vi "TrendPlot.vi"(6 "Zen Analytics in":refnum<class "Zen Analytics.lvclass">, 8 "error in (no error)":errorcluster, 9 "Graph Refference's":T2, 10 "IndexOfMeasurement":i32, 11 "Plot Cluster":T1) -> (0 "error out":errorcluster)   [LabVIEW 2019, in "Zen Analytics.lvlib" / "Zen Analytics.lvclass"]
uses:
  Zen Analytics.lvclass
  Dependency/GraphReff.ctl
  Dependency/Plot Cluster.ctl
types:
  T1 = typedef "Zen Analytics.lvlib/Zen Analytics.lvclass/Plot Cluster.ctl" = cluster{"Reduced 2D":dbl[][], "Start Index":i32, "No Of New Termnals":i32, "Top/Bottom":bool, "Values Inserted":i32, "Re-Initialised":bool, "Statistical params":string[][], "MeasurementInitializationData":cluster{"Measurement-ID":i32[], "Measurement Names":string[], "NominalValues":dbl[], "LSL":dbl[], "USL":dbl[], "LCL":dbl[], "UCL":dbl[]}, "MeasurementData":cluster{"Measurement ID":i32, "Measurement Name":string, "Nominal Values":dbl, "LSL":dbl, "USL":dbl, "LCL":dbl, "UCL":dbl}[], "ResultData2D":dbl[][], "PlotParameters":cluster{"Trend":cluster{"TrendPlotID":dbl, "PlotProperties":cluster{"FontName":string, "FontSize":dbl, "FontColor":string, "IsBold":bool, "IsItalic":bool, "PlotColor":string}}[], "Histogram":cluster{"HistogramPlotID":dbl, "PlotProperties":cluster{"FontName":string, "FontSize":dbl, "FontColor":string, "IsBold":bool, "IsItalic":bool, "PlotColor":string}}[], "BarPlot":cluster{"BarPlotID":dbl, "BarValuesID":dbl, "PlotProperties":cluster{"FontName":string, "FontSize":dbl, "IsBold":bool, "IsItalic":bool, "FontColor":string}, "Sectors":string[]}[], "PieChart":cluster{"PieChartID":dbl, "PieChartValueID":dbl, "PlotProperties":cluster{"FontName":string, "FontSize":dbl, "IsBold":bool, "IsItalic":bool, "FontColor":string}, "Sectors":string[]}[]}}
  T2 = typedef "Zen Analytics.lvlib/Zen Analytics.lvclass/GraphReff.ctl" = cluster{"HistgramGraph-reff":refnum<vi>[], "BarGraph-reff":refnum<vi>[], "PieGraph-reff":refnum<vi>[], "Lable-reff":refnum<vi>[], "TrendGraph-reff":refnum<vi>[], "CpCpkTable":refnum<vi>}
  T3 = cluster{"Measurement-ID":i32[], "Measurement Names":string[], "NominalValues":dbl[], "LSL":dbl[], "USL":dbl[], "LCL":dbl[], "UCL":dbl[]}
  T4 = cluster{"StartIndex":i32, "Index":i32, "TrendValue":dbl[][]}
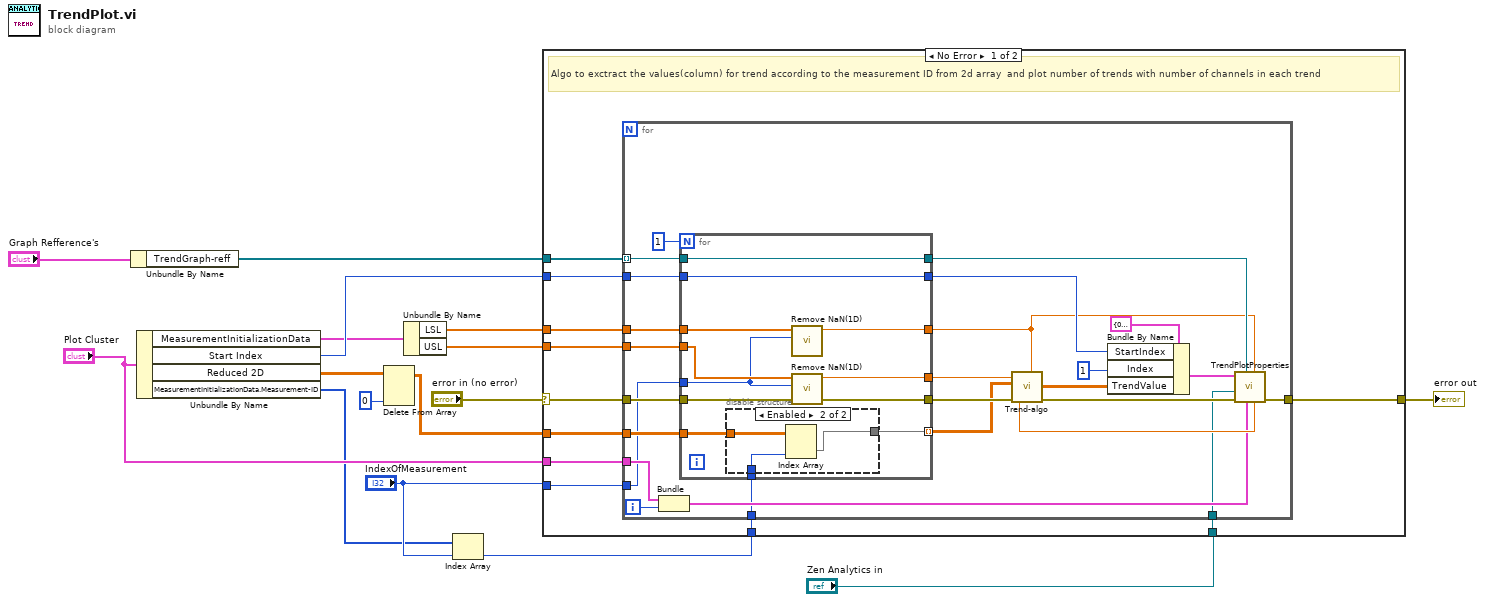
[diagram p0: block diagram]
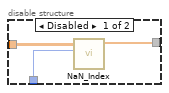
[diagram p2: hidden frame]
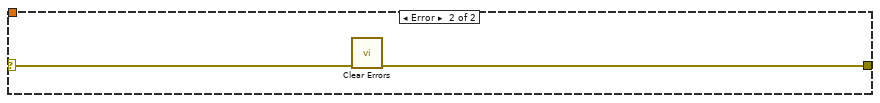
[diagram p3: hidden frame]
diagram:
  n1 = Unbundle By Name("Graph Refference's") -> ("TrendGraph-reff"=w15:refnum<vi>[])
  n2 = Unbundle By Name("Plot Cluster") -> ("MeasurementInitializationData"=w9:T3, "Start Index"=w12:i32, "Reduced 2D"=w8:dbl[][], "MeasurementInitializationData.Measurement-ID"=w3:i32[])
  n3 = Delete From Array(array=w8, index (col)=0 ("index")) -> (array with subset deleted=w5:dbl[][])  [unwired: 2 in, 1 out]
  n4 = Unbundle By Name(w9) -> ("LSL"=w13:dbl[], "USL"=w14:dbl[])
  n5 = Index Array(array=w3, index="IndexOfMeasurement") -> (element=w6:i32)
  n6 = case shown="No Error" "error in (no error)" {
    selector: "error in (no error)" -> [w20 w71]
    tunnel: [w23 w70] -> w2
    tunnel: w15 -> [w24 _]
    tunnel: w13 -> [w27 _]
    tunnel: w14 -> [w26 _]
    tunnel: w5 -> [w25 _]
    tunnel: w12 -> [w22 _]
    tunnel: "Plot Cluster" -> [w21 _]
    tunnel: "IndexOfMeasurement" -> [w19 _]
    tunnel: w6 -> [w18 _]
    tunnel: "Zen Analytics in" -> [w17 _]
    frame No Error {
      # "Algo to exctract the values(column) for trend according to the measurement ID from 2d array  and plot number of trends with number of channels in each trend"
      n7 = for {
        tunnel: w27 -> [w52]
        tunnel: w20 -> [w51]
        tunnel: w26 -> [w49]
        tunnel: w25 -> [w50]
        tunnel: w24 -> [w30] mode=indexing
        tunnel: [w35] -> w23
        tunnel: w22 -> [w44]
        tunnel: w21 -> [w37]
        tunnel: w19 -> [w29]
        tunnel: w18 -> [w31]
        tunnel: w17 -> [w28]
        i -> [w38]
        n8 = Bundle("Plot Cluster"=w37, w38) -> (w36:cluster{"Plot Cluster":T1, i32})  [unwired: 1 in]
        n9 = for {
          N: 1 -> [_]
          tunnel: w52 -> [w60]
          tunnel: w50 -> [w61]
          tunnel: w49 -> [w58]
          tunnel: w51 -> [w63]
          tunnel: [w55] -> w32 mode=indexing
          tunnel: [w63] -> w48
          tunnel: [w57] -> w39
          tunnel: [w59] -> w40
          tunnel: [w62] -> w41
          tunnel: w30 -> [w62]
          tunnel: [w56] -> w43
          tunnel: w44 -> [w56]
          tunnel: w31 -> [w54]
          tunnel: w29 -> [w53]
          n10 = disable-structure shown="Enabled" {
            disable-tunnel: w61 -> [w66 w69]
            disable-tunnel: [w65 w67] -> w55
            disable-tunnel: w54 -> [w64 w68]
            frame Disabled {
              n11 = call "NaN_Index.vi"("Index"=w64, "Input"=w66) -> ("Output"=w65:dbl[])  [unwired: 8 in, 1 out]
            }
            frame Enabled {
              n12 = Index Array(array=w69, index (col)=w68) -> (element=w67:dbl[])  [unwired: 1 in]
            }
          }
          n13 = call "Remove NaN(1D).vi"("Index"=w53, "Input"=w60) -> ("Numeric"=w59:dbl)  [unwired: 9 in]
          n14 = call "Remove NaN(1D).vi"("Index"=w53, "Input"=w58) -> ("Numeric"=w57:dbl)  [unwired: 9 in]
        }
        n15 = call "Trend-algo.vi"("LSL"=w40, "USL"=w39, "error in (no error)"=w48, "ReducedOutputData"=w32) -> ("error out"=w34:errorcluster, "OutputData-Trend"=w46:dbl[][])  [unwired: 6 in]
        n16 = Bundle By Name(cluster=T4 {"StartIndex"=0, "Index"=0, "TrendValue"=[]} ("Measurement-Summary 2"), "StartIndex"=w43, "Index"=1, "TrendValue"=w46) -> (w42:T4)
        n17 = call "TrendPlotProperties.vi"("UCL"=w39, "LCL"=w40, "Plot Cluster Index out"=w36, "TrendReff"=w41, "error in (no error)"=w34, "Zen Analytics in"=w28, "TrendValues"=w42) -> ("error out"=w35:errorcluster)  [unwired: 4 in]
      }
    }
    frame Error {
      n18 = call <vilib>:"Clear Errors.vi"("error in (no error)"=w71) -> ("error out"=w70:errorcluster)  [unwired: 5 in, 1 out]
    }
  }
  "error out" <- w2
